vi "createRegisters.vi"() -> (4 "ControllerRegisters":T1={"Parameters"="Parameters", "VDCLinkToP_PISettings"="Range", "ID_to_VD_PISettings"="gains", "IQ_to_VQ_PISettings"="Setpoints"})   [LabVIEW 2017, in "ActiveFrontEnd.lvlib"]
uses:
  ActiveFrontEnd.lvlib
  ControllerRegisters.ctl
  <vilib>/rvi/DataTransferAndStorage/Container/Common/niFpgaContainerGetUniqueNameForEmu.vi
  <vilib>/rvi/DataTransferAndStorage/Container/Common/niFpgaContainerSetEmuInfo.vi
  <vilib>/rvi/eio/common/nirviEmuReportErrorAndStop.vi
  <vilib>/rvi/LocalResourceManager/LocalResourceManager.xnode
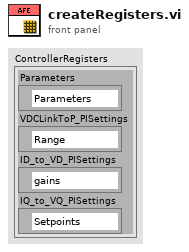
[diagram p1: front panel]
types:
  T1 = typedef "ActiveFrontEnd.lvlib/ControllerRegisters.ctl" = cluster{"Parameters":refnum<k21>, "VDCLinkToP_PISettings":refnum<k21>, "ID_to_VD_PISettings":refnum<k21>, "IQ_to_VQ_PISettings":refnum<k21>}
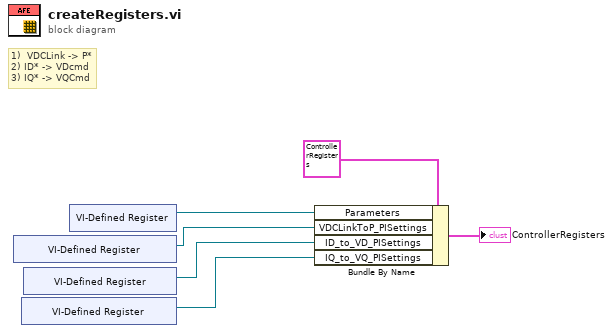
[diagram p0: block diagram]
diagram:
  # "1)  VDCLink -> P*\n2) ID* -> VDcmd\n3) IQ* -> VQCmd"
  n1 = xnode "VI-Defined Register"() -> ("Register Out"=w3:refnum<k21>)
  n2 = xnode "VI-Defined Register"() -> ("Register Out"=w1:refnum<k21>)
  n3 = xnode "VI-Defined Register"() -> ("Register Out"=w2:refnum<k21>)
  n4 = xnode "VI-Defined Register"() -> ("Register Out"=w4:refnum<k21>)
  n5 = Bundle By Name(cluster=T1 {"Parameters"="Parameters", "VDCLinkToP_PISettings"="Range", "ID_to_VD_PISettings"="gains", "IQ_to_VQ_PISettings"="Setpoints"}, "Parameters"=w4, "VDCLinkToP_PISettings"=w3, "ID_to_VD_PISettings"=w2, "IQ_to_VQ_PISettings"=w1) -> (→"ControllerRegisters":T1)
